vi "Dichroic Ratio.vi"(0 "Voltage":dbl, 5 "R":dbl, 7 "Correction Factor":dbl=2.9571 format="%#_13g", 9 "Ipar_ref":dbl=0.260692 format="%#_13g", 11 "Iperp_ref":dbl=0.145758 format="%#_13g") -> (4 "Dichroic Ratio":dbl)   [LabVIEW 2017, in "LD Reading.lvclass"]
uses:
  LD Reading.lvclass
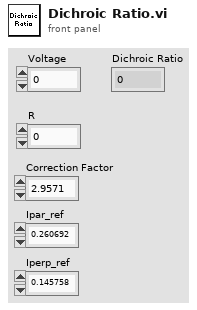
[diagram p1: front panel]
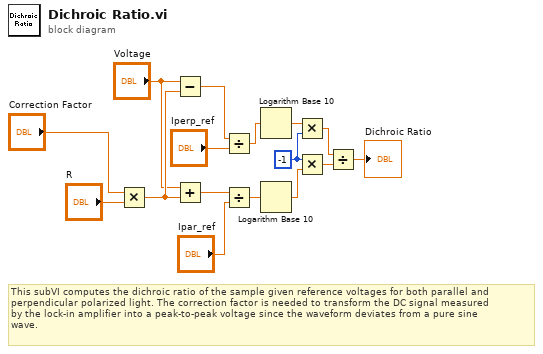
[diagram p0: block diagram]
diagram:
  w2 = -1
  # "This subVI computes the dichroic ratio of the sample given reference voltages for both parallel and \nperpendicular polarized light. The correction factor is needed to transform the DC signal measured \nby the lock-in amplifier into a peak-to-peak voltage since the waveform deviates from a pure sine \nwave."
  n1 = Multiply(x="Correction Factor", y="R") -> (x*y=w9:dbl)
  n2 = Subtract(x="Voltage", y=w9) -> (x-y=w13:dbl)
  n3 = Add(x="Voltage", y=w9) -> (x+y=w11:dbl)
  n4 = Divide(x=w13, y="Iperp_ref") -> (x/y=w14:dbl)
  n5 = Divide(x=w11, y="Ipar_ref") -> (x/y=w15:dbl)
  n6 = Logarithm Base 10(1:w14) -> (0:w1:dbl)
  n7 = Logarithm Base 10(1:w15) -> (0:w3:dbl)
  n8 = Multiply(x=w1, y=w2) -> (x*y=w5:dbl)
  n9 = Multiply(x=w2, y=w3) -> (x*y=w4:dbl)
  n10 = Divide(x=w5, y=w4) -> (x/y=→"Dichroic Ratio":dbl)
